vi "Read Element of Sections.vi"(8 "error in (no error)":errorcluster, 10 "index":i32, 11 "Configuration in":refnum<class "Configuration.lvclass">) -> (0 "error out":errorcluster, 2 "Section":refnum<class "Section.lvclass">, 3 "Configuration out":refnum<class "Configuration.lvclass">)   [LabVIEW 2013, in "Configuration.lvlib" / "Configuration.lvclass"]
doc: "Read section by index from class private data."
uses:
  Configuration.lvclass
  Section/Section.lvclass
  Configuration.lvclass/Configuration.ctl
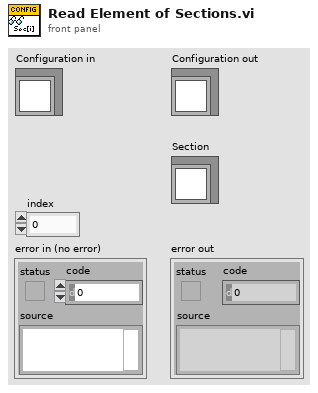
[diagram p1: front panel]
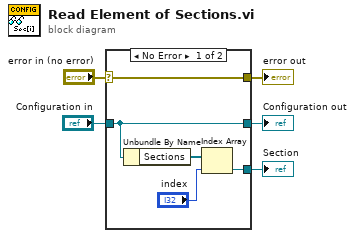
[diagram p0: block diagram]
diagram:
  n1 = case shown="No Error" "error in (no error)" {
    selector: "error in (no error)" -> [w10 w11]
    tunnel: [w10 w11] -> w4
    tunnel: [w9 w12] -> w2
    tunnel: "Configuration in" -> [w9 w12]
    tunnel: [w6 _] -> w1
    frame No Error {
      n2 = Unbundle By Name(w9) -> ("Sections"=w8:refnum<class "Section.lvclass">[])
      n3 = Index Array(array=w8, index="index") -> (element=w6:refnum<class "Section.lvclass">)
    }
    frame Error {
    }
  }
  "error out" <- w4
  "Configuration out" <- w2
  "Section" <- w1
